vi "emi_Bool Changed.vi"(7 "x":bool) -> (6 "Rising":bool, 8 "changed":bool, 10 "Falling":bool)   [LabVIEW 2011]
doc: "Monitors a bool, indicateing change, and wheter it was rising or falling. \n\nFirst call will always give out false on all outputs, asuming the previous is the same as the first.\n\nreentrant Subroutine."
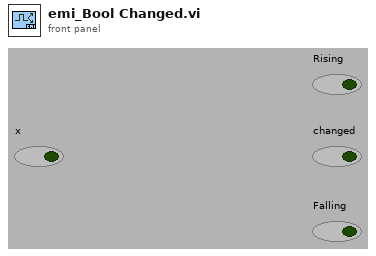
[diagram p1: front panel]
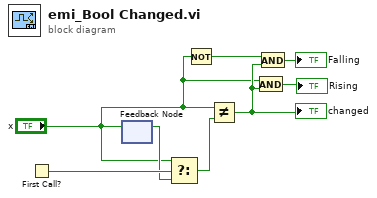
[diagram p0: block diagram]
diagram:
  n1 = First Call?() -> (First Call?: T/F=w8:bool)
  n2 = feedback-in #1("x") -> ()
  n3 = feedback #1() -> (w7:bool)  [unwired: 1 in]
  n4 = Select(t="x", s=w8, f=w7) -> (s? t:f=w6:bool)
  n5 = Not(x="x") -> (.not. x?=w3:bool)
  n6 = Not Equal?(x="x", y=w6) -> (x != y?=w2:bool)
  "changed" <- w2
  n7 = And(x="x", y=w2) -> (x .and. y?=→"Rising":bool)
  n8 = And(x=w3, y=w2) -> (x .and. y?=→"Falling":bool)
